vi "_getAllProperties.vi"(8 "error in (no error)":errorcluster, 11 "storage refnum":refnum<k20>) -> (0 "error out":errorcluster, 2 "property name value":string[][](array[string]), 3 "storage refnum out":refnum<k20>)   [LabVIEW 2020]
uses:
  <vilib>/Platform/storage/Storage.llb/Get Property (String).vi
  <vilib>/Platform/storage/Storage.llb/Get Property (Time Stamp).vi
  <vilib>/Platform/storage/Storage.llb/Get Property (Enum).vi
  <vilib>/Platform/storage/Storage.llb/Get Property (I32).vi
  <vilib>/Platform/storage/Storage.llb/Get Property (DBL).vi
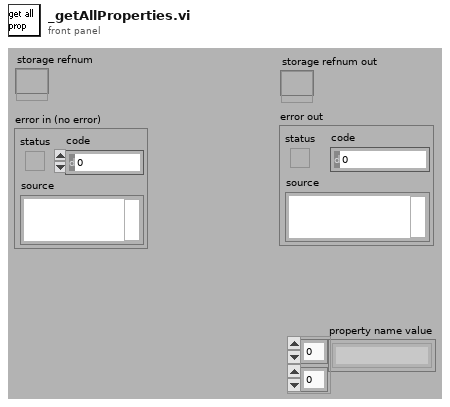
[diagram p1: front panel]
types:
  T1 = typedef "usiProperty.ctl" = cluster{"object type":T2, "property name":string, "data type":T3}
  T2 = typedef "usiObjectType.ctl" = enum16{"File", "Channel Group", "Channel", "Unknown"}
  T3 = typedef "usiDataType.ctl" = enum16{"eNoTypeUsi", "eInt8Usi", "eInt16Usi", "eInt32Usi", "eInt64Usi", "eUInt8Usi", "eUInt16Usi", "eUInt32Usi", "eUInt64Usi", "eFloat32Usi", "eFloat64Usi", "- 0", "- 1", "- 2", "- 3", "- 4", "- 5", "- 6", "- 7", "- 8", "- 9", "eString8Usi", "eString16Usi", "eStringUsi", "eEnumUsi", "- 10", "- 11", "- 12", "- 13", "- 14", "eTimeUsi", "- 15", "- 16", "- 17", "- 18", "- 19", "- 20", "- 21", "- 22", "- 23", "eInstanceUsi", "eStoreUsi"}
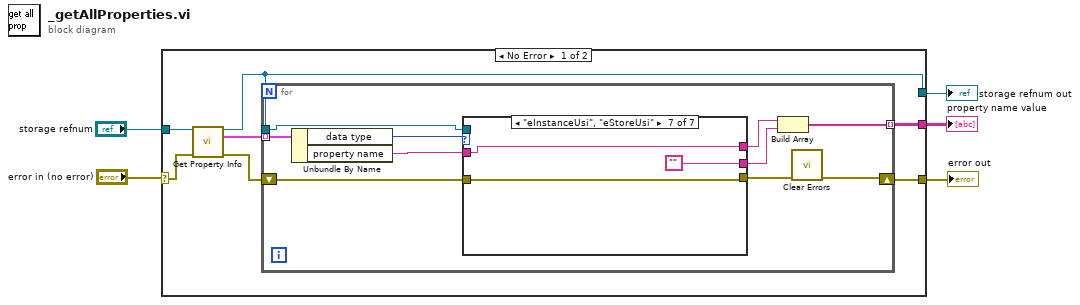
[diagram p0: block diagram]
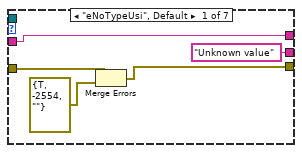
[diagram p2: hidden frame]
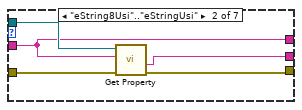
[diagram p3: hidden frame]
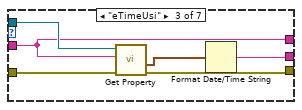
[diagram p4: hidden frame]
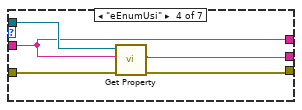
[diagram p5: hidden frame]
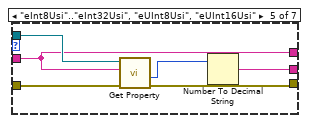
[diagram p6: hidden frame]
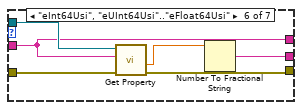
[diagram p7: hidden frame]
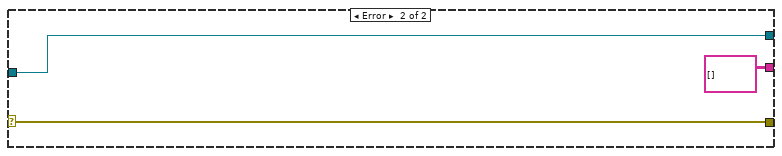
[diagram p8: hidden frame]
diagram:
  n1 = case shown="No Error" "error in (no error)" {
    selector: "error in (no error)" -> [w6 w59]
    tunnel: "storage refnum" -> [w12 w61]
    tunnel: [w10 w61] -> w4
    tunnel: [w8 string[][] []] -> w3
    tunnel: [w7 w59] -> w2
    frame No Error {
      n2 = call <vilib>:"Get Property Info.vi"("storage refnum"=w12, "error in (no error)"=w6) -> ("storage refnum out"=w10:refnum<k20>, "properties"=w11:T1[], "error out"=w9:errorcluster)  [unwired: 11 in]
      n3 = for {
        tunnel: w11 -> [w22] mode=indexing
        tunnel: w10 -> [w17]
        shift-right: [w14] -> w7
        shift-left: w9 -> [w20]
        tunnel: [w13] -> w8 mode=indexing
        n4 = Unbundle By Name(w22) -> ("data type"=w21:T3, "property name"=w19:string)
        n5 = case shown="\"eInstanceUsi\", \"eStoreUsi\"" w21 {
          tunnel: w20 -> [w27 w32 w38 w43 w49 w55 w58]
          tunnel: w19 -> [w24 w28 w35 w40 w46 w52 w56]
          tunnel: [w25 w31 w37 w42 w48 w54 w58] -> w18
          tunnel: ["Unknown value" ("Value") w30 w33 w39 w44 w51 ""] -> w15
          tunnel: w17 -> [_ w29 w36 w41 w47 w53 _]
          tunnel: [w24 w28 w35 w40 w46 w52 w56] -> w16
          frame "eNoTypeUsi", Default {
            n6 = Merge Errors(w27, errorcluster {"status"=TRUE, "code"=-2554, "source"=""} ("error in 2 (no error)")) -> (w25:errorcluster)
          }
          frame "eString8Usi".."eStringUsi" {
            n7 = call-poly <vilib>:"Get Property.vi"("error in (no error)"=w32, "Property name"=w28, "storage refnum"=w29) -> ("error out"=w31:errorcluster, "Value"=w30:string)  [unwired: 6 in, 1 out]
          }
          frame "eTimeUsi" {
            n8 = call-poly <vilib>:"Get Property.vi"("error in (no error)"=w38, "Property name"=w35, "storage refnum"=w36) -> ("error out"=w37:errorcluster, "Value"=w34:timestamp)  [unwired: 6 in, 1 out]
            n9 = Format Date/Time String(seconds (now)=w34) -> (date/time string=w33:string)  [unwired: 2 in]
          }
          frame "eEnumUsi" {
            n10 = call-poly <vilib>:"Get Property.vi"("error in (no error)"=w43, "Property name"=w40, "storage refnum"=w41) -> ("error out"=w42:errorcluster, "String"=w39:string)  [unwired: 5 in, 2 out]
          }
          frame "eInt8Usi".."eInt32Usi", "eUInt8Usi", "eUInt16Usi" {
            n11 = call-poly <vilib>:"Get Property.vi"("error in (no error)"=w49, "Property name"=w46, "storage refnum"=w47) -> ("error out"=w48:errorcluster, "Value"=w45:i32)  [unwired: 6 in, 1 out]
            n12 = Number To Decimal String(number=w45) -> (decimal integer string=w44:string)  [unwired: 1 in]
          }
          frame "eInt64Usi", "eUInt64Usi".."eFloat64Usi" {
            n13 = call-poly <vilib>:"Get Property.vi"("error in (no error)"=w55, "Property name"=w52, "storage refnum"=w53) -> ("error out"=w54:errorcluster, "Value"=w50:dbl)  [unwired: 6 in, 1 out]
            n14 = Number To Fractional String(number=w50) -> (F-format string=w51:string)  [unwired: 3 in]
          }
          frame "eInstanceUsi", "eStoreUsi" {
          }
        }
        n15 = Build Array(w16, w15) -> (w13:string[])
        n16 = call <vilib>:"Clear Errors.vi"("error in (no error)"=w18) -> ("error out"=w14:errorcluster)  [unwired: 5 in, 1 out]
      }
    }
    frame Error {
    }
  }
  "property name value" <- w3
  "error out" <- w2
  "storage refnum out" <- w4
